vi "DSF.Transceiver.GE Reflective Memory.Initialize Transfer Group Parameters.vi"(8 "error in (no error)":errorcluster, 10 "Transfer Groups Configurations":refnum<class "DSF.Shared.Configuration.Transfer Group.lvclass">[](array[class]), 11 "DSF GE Reflective Memory Transceiver in":refnum<class "DSF.Transceiver.GE Reflective Memory.lvclass">) -> (0 "error out":errorcluster, 3 "DSF GE Reflective Memory Transceiver out":refnum<class "DSF.Transceiver.GE Reflective Memory.lvclass">)   [LabVIEW 2017, in "DSF.Transceiver.GE Reflective Memory.lvlib" / "DSF.Transceiver.GE Reflective Memory.lvclass"]
uses:
  DSF.Transceiver.GE Reflective Memory.lvclass
  DSF Core/Built/Engine/DSF.Engine.lvlibp/Shared/Classes/Transfer Group/DSF.Shared.Configuration.Transfer Group.lvclass
  DSF.Transceiver.GE Reflective Memory.Transfer Group Parameters.ctl
  <vilib>/NI/GE Reflective Memory Driver/Typedefs/GE 5565PIORC.Typedef.DMA Transfer Spec.ctl
  <vilib>/NI/GE Reflective Memory Driver/Typedefs/GE 5565PIORC.Typedef.DMA Block Descriptor.ctl
  <vilib>/NI/GE Reflective Memory Driver/Typedefs/GE 5565PIORC.Typedef.DMA Block Descriptor Params.ctl
  DSF.Transceiver.GE Reflective Memory.lvclass/DSF.Transceiver.GE Reflective Memory.ctl
  <vilib>/NI/GE Reflective Memory Driver/GE 5565PIORC.lvclass/GE 5565PIORC.ctl
  <vilib>/NI/GE Reflective Memory Driver/Methods/GE 5565PIORC.DMA.Create Transfer (Block).vi
  <vilib>/NI/GE Reflective Memory Driver/Methods/GE 5565PIORC.DMA.Create Transfer (Scatter-Gather).vi
  <vilib>/NI/GE Reflective Memory Driver/Methods/GE 5565PIORC.DMA.Size.vi
  <vilib>/NI/GE Reflective Memory Driver/Methods/GE 5565PIORC.Round Up to Nearest 8.vi
  <vilib>/NI/GE Reflective Memory Driver/Methods/GE 5565PIORC.Round Up to Nearest 16.vi
  <vilib>/NI/GE Reflective Memory Driver/GE 5565PIORC.lvclass
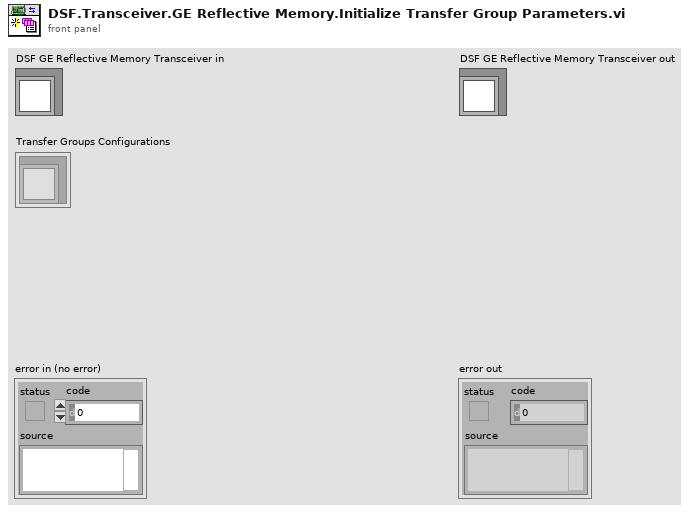
[diagram p1: front panel]
types:
  T1 = typedef "DSF.Transceiver.GE Reflective Memory.lvlib/DSF.Transceiver.GE Reflective Memory.lvclass/DSF.Transceiver.GE Reflective Memory.Transfer Group Parameters.ctl" = cluster{"DMA Transfer Specs":T2[]}
  T2 = typedef "GE 5565PIORC.lvclass/GE 5565PIORC.Typedef.DMA Transfer Spec.ctl" = cluster{"RFM offset":u32, "Block Descriptors":T3[]}
  T3 = typedef "GE 5565PIORC.lvclass/GE 5565PIORC.Typedef.DMA Block Descriptor.ctl" = cluster{"descriptor ptr (VISA)":u32, "descriptor ptr (RFM)":u32, "descriptor size":u32, "descriptor params":T4}
  T4 = typedef "GE 5565PIORC.lvclass/GE 5565PIORC.Typedef.DMA Block Descriptor Params.ctl" = cluster{"data ptr (lower)":u32, "data ptr (upper)":u32, "data size":u32, "next descriptor ptr":u32}
  T5 = typedef "DSF.Transceiver.GE Reflective Memory.lvlib/DSF.Transceiver.GE Reflective Memory.lvclass/DSF.Transceiver.GE Reflective Memory.Transfer Parameters.ctl" = cluster{"offset":u32, "size":u32}
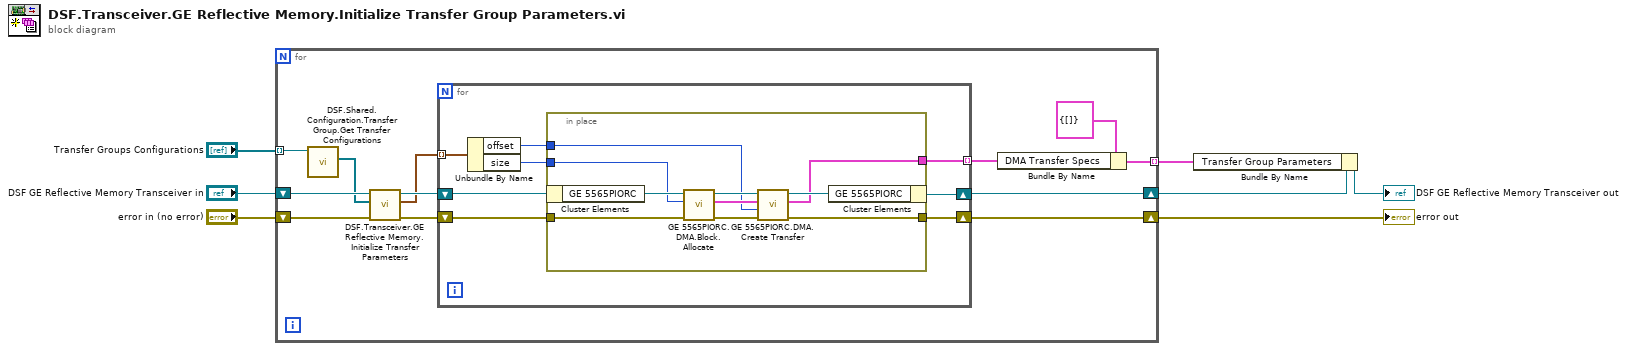
[diagram p0: block diagram]
diagram:
  n1 = for {
    tunnel: "Transfer Groups Configurations" -> [w17] mode=indexing
    shift-right: [w11] -> w3
    shift-left: "DSF GE Reflective Memory Transceiver in" -> [w15]
    shift-right: [w10] -> w4
    shift-left: "error in (no error)" -> [w16]
    tunnel: [w18] -> w1 mode=indexing
    n2 = call "DSF.Shared.Configuration.Transfer Group.Get Transfer Configurations.vi"("Transfer Group Configuration in"=w17) -> ("Transfer Configurations"=w8:refnum<class "DSF.Shared.Configuration.Transfer.lvclass">[])  [unwired: 9 in, 1 out]
    n3 = call "DSF.Transceiver.GE Reflective Memory.Initialize Transfer Parameters.vi"("error in (no error)"=w16, "Transfer Configurations"=w8, "DSF GE Reflective Memory Transceiver in"=w15) -> ("error out"=w14:errorcluster, "Transfers Parameters"=w12:T5[], "DSF GE Reflective Memory Transceiver out"=w13:refnum<class "DSF.Transceiver.GE Reflective Memory.lvclass">)  [unwired: 6 in]
    n4 = for {
      tunnel: w12 -> [w25] mode=indexing
      shift-right: [w21] -> w10
      shift-left: w14 -> [w27]
      tunnel: [w22] -> w9 mode=indexing
      shift-right: [w20] -> w11
      shift-left: w13 -> [w26]
      n5 = Unbundle By Name(w25) -> ("offset"=w23:u32, "size"=w24:u32)
      n6 = in-place {
        in-place-border: [w36] -> w21
        in-place-border: [w30] -> w22
        in-place-border: w27 -> [w32]
        in-place-border: w24 -> [w31]
        in-place-border: w23 -> [w28]
        n7 = in-place-cluster #1(w26) -> ("GE 5565PIORC"=w34:refnum<class "GE 5565PIORC.lvclass">)
        n8 = call <vilib>:"GE 5565PIORC.DMA.Block.Allocate.vi"("error in (no error)"=w32, "size in bytes"=w31, "GE 5565PIORC in"=w34) -> ("error out"=w37:errorcluster, "Block Descriptor"=w29:T3, "GE 5565PIORC out"=w35:refnum<class "GE 5565PIORC.lvclass">)  [unwired: 6 in]
        n9 = call-poly <vilib>:"GE 5565PIORC.DMA.Create Transfer.vi"("error in (no error)"=w37, "RFM offset"=w28, "Block Descriptor"=w29, "GE 5565PIORC in"=w35) -> ("error out"=w36:errorcluster, "DMA Transfer Spec"=w30:T2, "GE 5565PIORC out"=w33:refnum<class "GE 5565PIORC.lvclass">)  [unwired: 4 in, 1 out]
        n10 = in-place-cluster #1("GE 5565PIORC"=w33) -> (w20:refnum<class "DSF.Transceiver.GE Reflective Memory.lvclass">)
      }
    }
    n11 = Bundle By Name(cluster=T1 {"DMA Transfer Specs"=[]} ("Transfer Group Parameters"), "DMA Transfer Specs"=w9) -> (w18:T1)
  }
  "error out" <- w4
  n12 = Bundle By Name(cluster=w3, "Transfer Group Parameters"=w1) -> (→"DSF GE Reflective Memory Transceiver out":refnum<class "DSF.Transceiver.GE Reflective Memory.lvclass">)
